vi "RecVOR _Ori.vi"() -> ()   [LabVIEW 2013]
uses:
  <vilib>/userdefined/High Color/IMAQdx.ctl
  <vilib>/vision/Avi1.llb/AviRefnum.ctl
  <vilib>/vision/driver/IMAQdx.llb/IMAQdx Attribute Visibility.ctl
  <vilib>/Instr/_visa.llb/VISA Configure Serial Port (Instr).vi
  <vilib>/DAQmx/read.llb/DAQmx Read (Digital Bool 1Line 1Point).vi
  <vilib>/DAQmx/read.llb/DAQmx Read (Counter U32 1Chan 1Samp).vi
  <vilib>/Utility/file.llb/Write To Spreadsheet File (DBL).vi
  <vilib>/vision/driver/NI_Vision_Acquisition_Software.lvlib
  <resource>/objmgr/imaqdx.rc
  <vilib>/vision/NI_Vision_Development_Module.lvlib
panel:
  in  "Image Flip":u32(ring)=3 items=["Horizontal Flip", "Vertical Flip", "Central Flip", "No Flip"]
  in  "Attribute Name":u32(ring) items=["CameraAttributes::Brightness::Mode", "CameraAttributes::Brightness::Value", "CameraAttributes::Exposure::Mode", "CameraAttributes::Exposure::Value", "CameraAttributes::Gain::Mode", "CameraAttributes::Gain::Value", "CameraAttributes::Gamma::Mode", "CameraAttributes::Gamma::Value", "CameraAttributes::Hue::Mode", "CameraAttributes::Hue::Value", "CameraAttributes::Pan::Mode", "CameraAttributes::Pan::Value", "CameraAttributes::Saturation::Mode", "CameraAttributes::Saturation::Value", "CameraAttributes::Sharpness::Mode", "CameraAttributes::Sharpness::Value", "CameraAttributes::Tilt::Mode", "CameraAttributes::Tilt::Value"]
  in  "Set":bool
  in  "Attribute Value":string
  in  "VISA resource name":refnum<visa-resource-name>="COM3"
  out "Waveform Chart 2":cluster{dbl, dbl}(graph)
  out "Start RecTime":timestamp
  out "Avi Refnum":T1
  out "Elapsed Time":dbl
  out "Frame Num":dbl
  in  "Codec:":string(combo)="Microsoft Video 1"
  out "Rec File Path:":path
  in  "Recording":bool
  in  "Camera Name:":T2="cam0"
  in  "stop":bool
  in  "OpenCam":bool
  out "Frame Rate":dbl(knob) scale=0.0..120.0
  in  "Tab Control":enum32{"Alignment", "Rotator"}(tab)
  out "Alignment":bool
  in  "BCGT":T3={"Brightness"=171.0, "Contrast"=89.0, "Gamma"=2.0, "Threshold_Low"=0.0, "Threshold_High"=255.0} {"Threshold_High" min=0.0 max=255.0 step=1.0 scale=0.0..255.0; "Threshold_Low" min=0 max=255 step=1 scale=0.0..255.0 scale format="%.2f"; "Gamma" min=0.1 max=10 step=0.01 scale=0.1..10.0 scale format="%.1f"; "Contrast" min=1 max=89 step=0.1 scale=0.0..89.0 scale format="%.2f"; "Brightness" min=0 max=255 step=1 scale=0.0..255.0 scale format="%.2f"}
  out "Number of Particles":i32
  out "Distances":sgl[](array[numeric]) format="%.4f"
  out "Array":cluster{"Numeric":dbl, "Numeric":dbl}[](array[cluster])
  out "Image 2":T4(plugin-control)
  out "Degree/sec":dbl(knob) scale=-105.0..105.0
  out "EMST":bool
  out "SVON":bool=TRUE
  in  "Select Mode":T5(ring)
  out "Received Data":string
  out "Transmit Data":string
  in  "Sent":bool
  in  "task/channels in":refnum<k21>="position"
  in  "task/channels in 2":refnum<k21>="dir"
  in  "task/channels in 3":refnum<k21>="dir_vel"
  out "Angle Position":dbl(knob)
  in  "Listbox":i32(listbox)
  in  "Add":bool
  in  "Time":dbl
  in  "Stop":bool
  out "Image":T4(plugin-control)
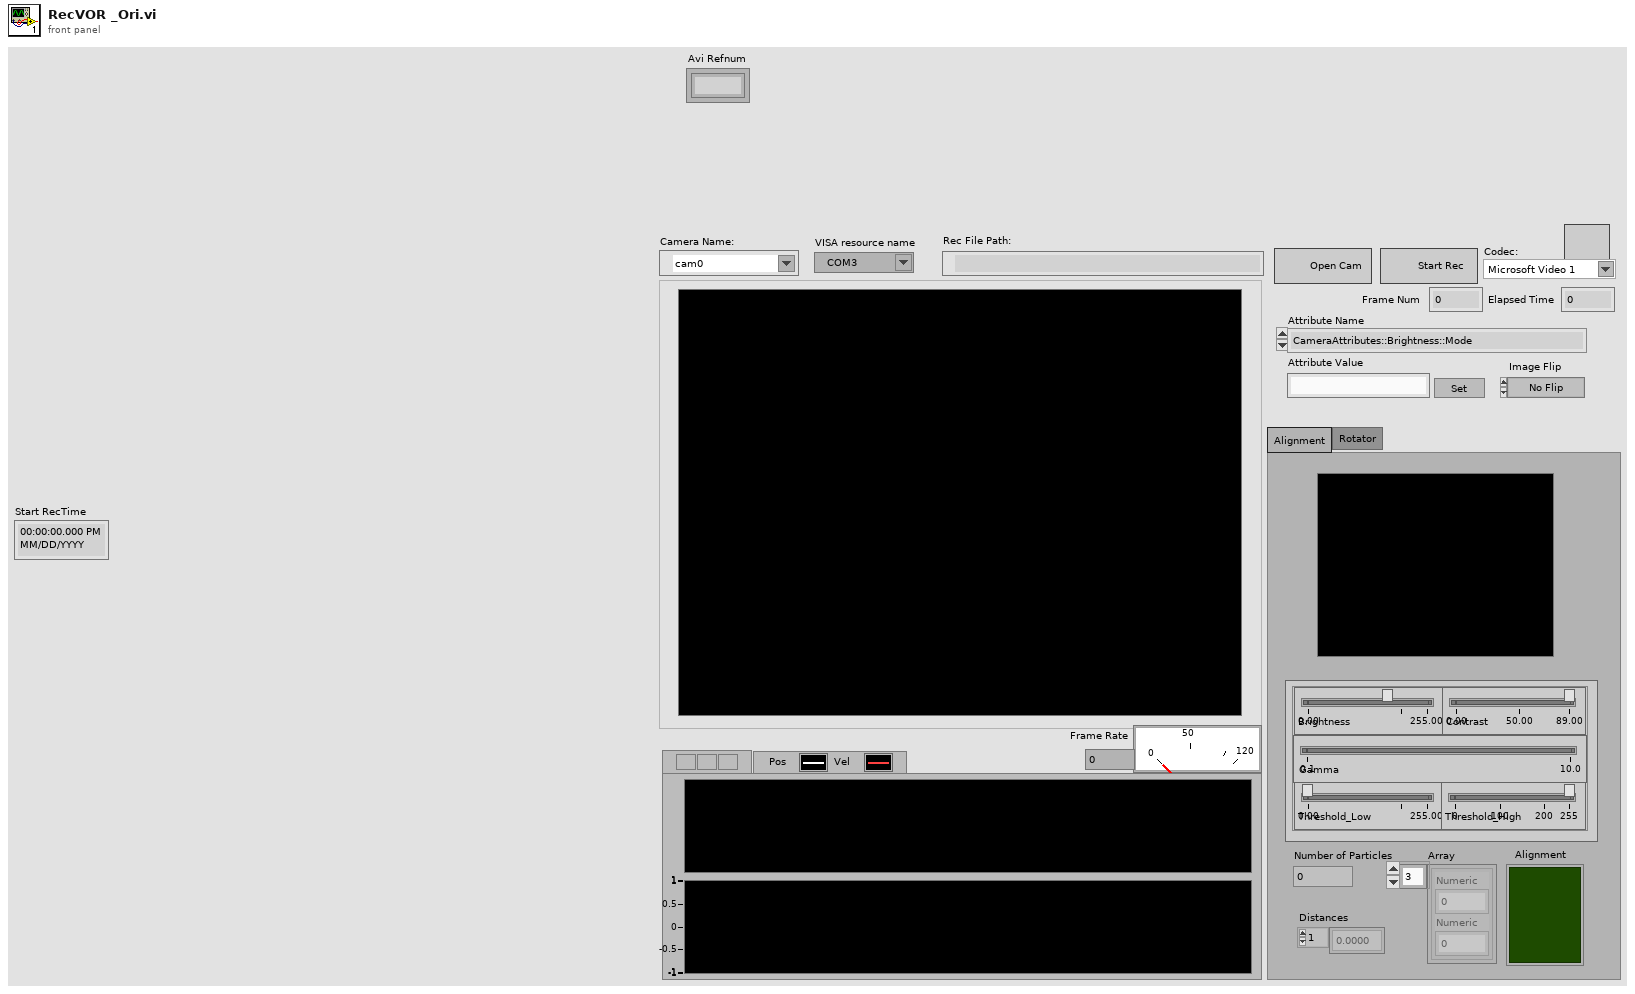
[diagram p1: front panel]
types:
  T1 = typedef "AviRefnum.ctl" = refnum<k1>
  T2 = typedef "IMAQdx.ctl" = refnum<k21>
  T3 = cluster{"Brightness":sgl, "Contrast":sgl, "Gamma":sgl, "Threshold_Low":sgl, "Threshold_High":dbl}
  T4 = typedef "IMAQ Image.ctl" = refnum<image>
  T5 = enum16{"SVON OFF", "SVON ON", "EMST OFF", "EMST ON", "15 degree, 0.1Hz", "15 degree, 0.2Hz", "15 degree, 0.5Hz", "15 degree, 1Hz", "15 degree, 2Hz", "15 degree, 4Hz", "15 degree, 6Hz", "15 degree, 8Hz", "15 degree, 10Hz", "30 degree, 0.1Hz", "30 degree, 0.2Hz", "30 degree, 0.5Hz", "30 degree, 1Hz", "30 degree, 2Hz", "30 degree, 4Hz", "30 degree, 6Hz", "30 degree, 8Hz", "30 degree, 10Hz", "60 degree, 0.1Hz", "60 degree, 0.2Hz", "60 degree, 0.5Hz", "60 degree, 1Hz", "60 degree, 2Hz", "60 degree, 4Hz", "60 degree, 6Hz", "60 degree, 8Hz", "100 degree, 0.1Hz", "100 degree, 0.2Hz", "100 degree, 0.5Hz", "100 degree, 1Hz"}
  T6 = enum8{"Enabled", "Disabled", "Disabled and Grayed Out"}
  T7 = enum16{"Calvar3Open", "CalDataOpen", "CalGrpOpen", "AddAvg", "RmvAvg", "CalCalvar", "AddVar", "SaveVar", "Up", "Dn", "Del"}
  T8 = typedef "NI_Vision_Acquisition_Software.lvlib/IMAQdx Attribute Visibility.ctl" = enum32{"Simple", "Intermediate", "Advanced"}
  T9 = typedef "NI_Vision_Acquisition_Software.lvlib/IMAQdx Attribute Type.ctl" = enum32{"U32", "I64", "DBL", "String", "Enum", "Bool", "Command"}
  T10 = cluster{"Attribute Type":T9, "Readable":bool, "Writable":bool, "Attribute Name":string}[]
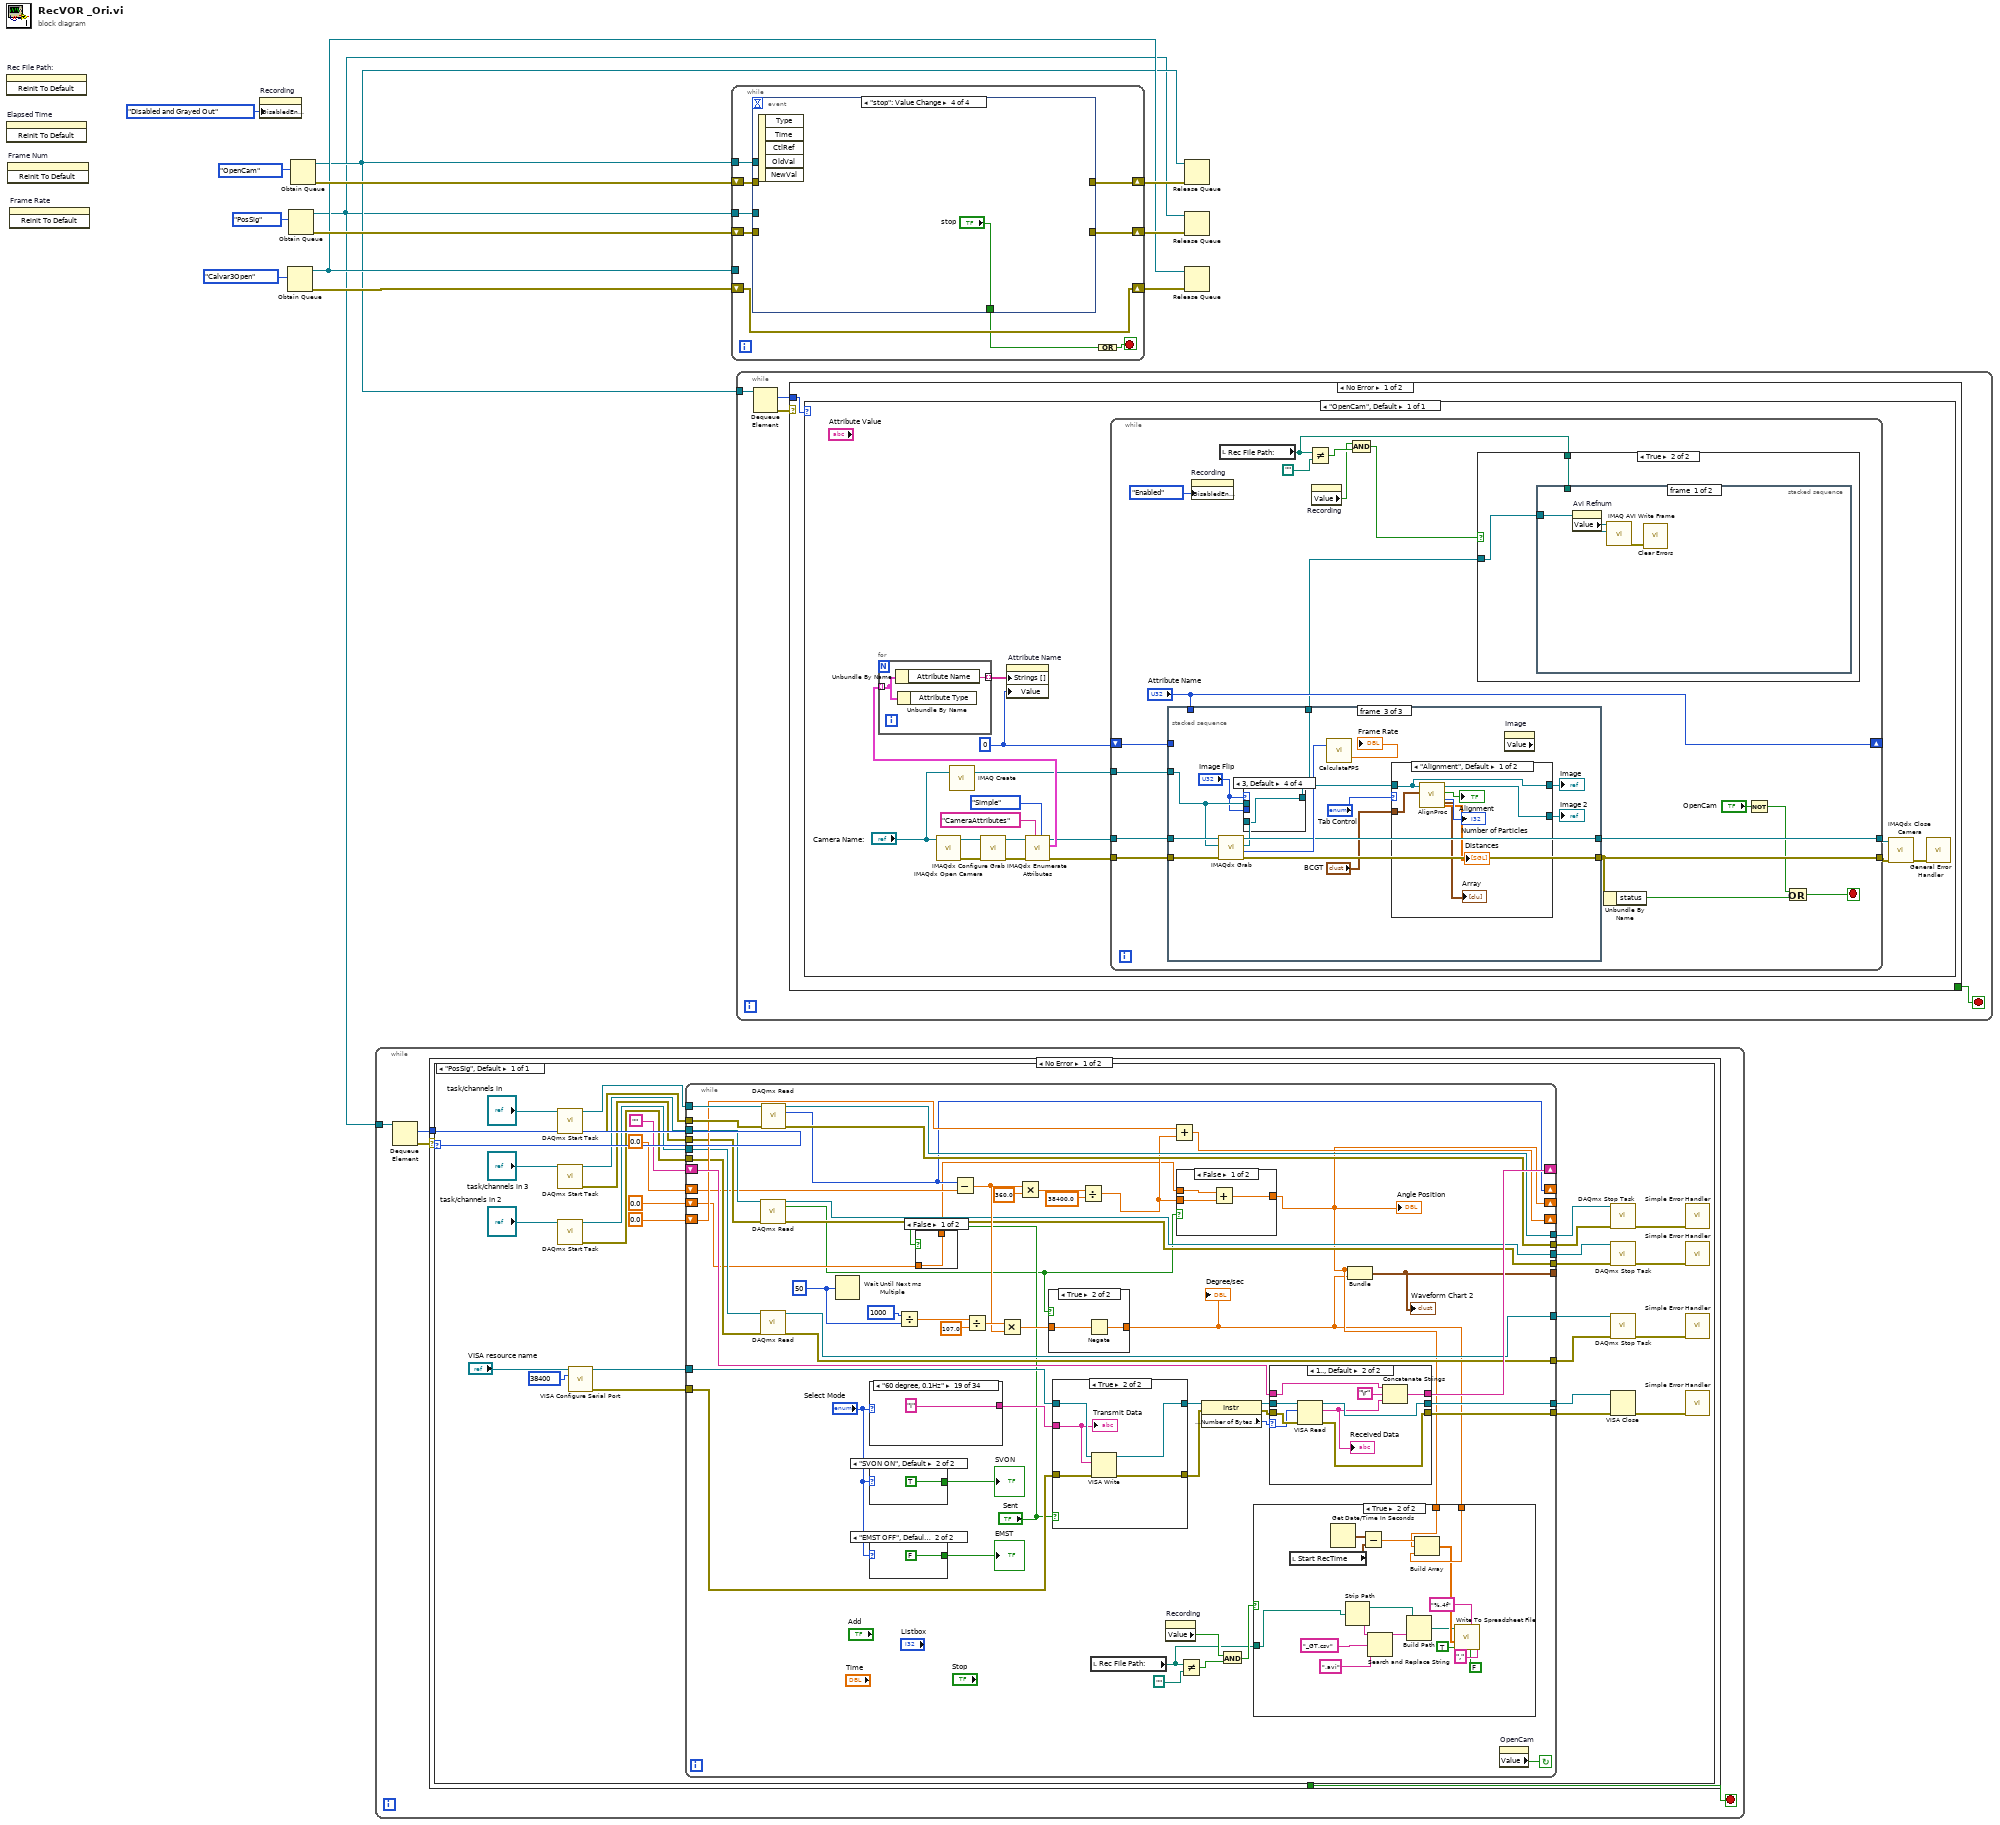
[diagram p0: block diagram]
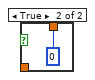
[diagram p3: hidden frame]
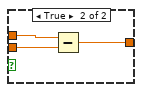
[diagram p5: hidden frame]
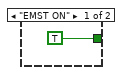
[diagram p6: hidden frame]
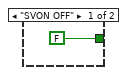
[diagram p7: hidden frame]
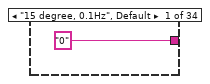
[diagram p8: hidden frame]
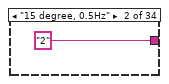
[diagram p9: hidden frame]
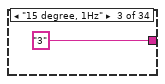
[diagram p10: hidden frame]
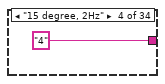
[diagram p11: hidden frame]
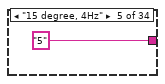
[diagram p12: hidden frame]
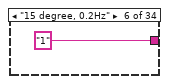
[diagram p13: hidden frame]
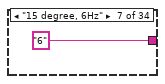
[diagram p14: hidden frame]
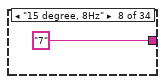
[diagram p15: hidden frame]
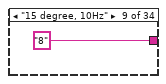
[diagram p16: hidden frame]
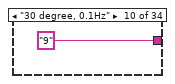
[diagram p17: hidden frame]
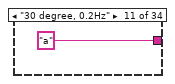
[diagram p18: hidden frame]
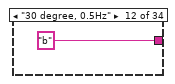
[diagram p19: hidden frame]
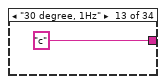
[diagram p20: hidden frame]
diagram:
  n1 = invoke on="Rec File Path:" class="Path" method="Reinit To Default"() -> ()  [unwired: 3 in, 3 out]
  n2 = invoke on="Elapsed Time" class="DigNum (strict)" method="Reinit To Default"() -> ()  [unwired: 3 in, 3 out]
  n3 = invoke on="Frame Num" class="DigNum (strict)" method="Reinit To Default"() -> ()  [unwired: 3 in, 3 out]
  n4 = invoke on="Frame Rate" class="Knob (strict)" method="Reinit To Default"() -> ()  [unwired: 3 in, 3 out]
  n5 = property on="Recording" class="Bool (strict)"("DisabledEnum"=T6."Disabled and Grayed Out" ("Disabled")) -> ()  [unwired: 2 in, 2 out]
  n6 = Obtain Queue(element data type=T7."Calvar3Open" ("Enum")) -> (queue out=w4:refnum<queue>, error out=w9:errorcluster)  [unwired: 4 in, 1 out]
  n7 = Obtain Queue(element data type=enum16{"PosSig"}."PosSig" ("Enum")) -> (queue out=w2:refnum<queue>, error out=w10:errorcluster)  [unwired: 4 in, 1 out]
  n8 = Obtain Queue(element data type=enum16{"OpenCam"}."OpenCam" ("Enum")) -> (queue out=w3:refnum<queue>, error out=w12:errorcluster)  [unwired: 4 in, 1 out]
  n9 = while {
    tunnel: w2 -> [w17]
    stop <- w15 stop-if-true
    n10 = Dequeue Element(queue=w17) -> (element=w14:enum16{"PosSig"}, error out=w16:errorcluster)  [unwired: 2 in, 2 out]
    n11 = case shown="No Error" w16 {
      tunnel: [_ TRUE] -> w15
      tunnel: w14 -> [w18 _]
      frame No Error {
        n12 = case shown="\"PosSig\", Default" w18 {
          frame "PosSig", Default {
            n13 = call <vilib>:"DAQmx Start Task.vi"("task/channels in"="task/channels in") -> ("task out"=w40:refnum<k21>, "error out"=w35:errorcluster)  [unwired: 13 in]
            n14 = call <vilib>:"DAQmx Start Task.vi"("task/channels in"="task/channels in 3") -> ("task out"=w24:refnum<k21>, "error out"=w23:errorcluster)  [unwired: 13 in]
            n15 = call <vilib>:"DAQmx Start Task.vi"("task/channels in"="task/channels in 2") -> ("task out"=w31:refnum<k21>, "error out"=w30:errorcluster)  [unwired: 13 in]
            n16 = call-poly "VISA Configure Serial Port"("VISA resource name"="VISA resource name", "baud rate (9600)"=u32 38400) -> ("VISA resource name out"=w44:refnum<visa-resource-name>, "error out"=w43:errorcluster)  [unwired: 12 in]
            n17 = while {
              tunnel: w43 -> [w101]
              tunnel: w44 -> [w102]
              shift-left: "" -> [w93]
              shift-right: [w92] -> _
              tunnel: [w95] -> w46
              tunnel: [w94] -> w47
              tunnel: [w87] -> w41
              tunnel: w40 -> [w86]
              tunnel: w35 -> [w85]
              tunnel: [w84] -> w39
              shift-right: [w75] -> _
              shift-left: 0.0 ("data") -> [w60]
              shift-right: [w74] -> _
              shift-left: 0.0 -> [w80]
              tunnel: w31 -> [w79]
              tunnel: w30 -> [w78]
              tunnel: [w77] -> w29
              tunnel: [w76] -> w28
              shift-right: [w54] -> _
              shift-left: 0.0 -> [w59]
              tunnel: [w56] -> _
              tunnel: w24 -> [w66]
              tunnel: w23 -> [w65]
              tunnel: [w63] -> w21
              tunnel: [w62] -> w20
              stop <- w57 continue-if-true
              w73 = u32 50 ("millisecond multiple")
              n18 = call-poly <vilib>:"DAQmx Read.vi"("task/channels in"=w66, "error in"=w65) -> ("task out"=w62:refnum<k21>, "data"=w55:bool, "error out"=w63:errorcluster)  [unwired: 11 in]
              n19 = call-poly <vilib>:"DAQmx Read.vi"("task/channels in"=w79, "error in"=w78) -> ("task out"=w76:refnum<k21>, "error out"=w77:errorcluster)  [unwired: 11 in, 1 out]
              n20 = call-poly <vilib>:"DAQmx Read.vi"("task/channels in"=w86, "error in"=w85) -> ("task out"=w84:refnum<k21>, "data"=w75:u32, "error out"=w87:errorcluster)  [unwired: 11 in]
              n21 = Wait Until Next ms Multiple(millisecond multiple=w73) -> ()  [unwired: 1 out]
              n22 = case shown="\"60 degree, 0.1Hz\"" "Select Mode" {
                tunnel: ["0" "2" "3" "4" "5" "1" "6" "7" "8" "9" "a" "b" "c" "d" "e" "f" "g" "h" "i" "j" "k" "l" "m" "n" "o" "p" "r" "t" "u" "v" "q" "z" "s" "w"] -> w91
                frame "15 degree, 0.1Hz", Default {
                }
                frame "15 degree, 0.5Hz" {
                }
                frame "15 degree, 1Hz" {
                }
                frame "15 degree, 2Hz" {
                }
                frame "15 degree, 4Hz" {
                }
                frame "15 degree, 0.2Hz" {
                }
                frame "15 degree, 6Hz" {
                }
                frame "15 degree, 8Hz" {
                }
                frame "15 degree, 10Hz" {
                }
                frame "30 degree, 0.1Hz" {
                }
                frame "30 degree, 0.2Hz" {
                }
                frame "30 degree, 0.5Hz" {
                }
                frame "30 degree, 1Hz" {
                }
                frame "30 degree, 2Hz" {
                }
                frame "30 degree, 4Hz" {
                }
                frame "30 degree, 6Hz" {
                }
                frame "30 degree, 8Hz" {
                }
                frame "30 degree, 10Hz" {
                }
                frame "60 degree, 0.1Hz" {
                }
                frame "60 degree, 0.2Hz" {
                }
                frame "60 degree, 0.5Hz" {
                }
                frame "60 degree, 1Hz" {
                }
                frame "60 degree, 2Hz" {
                }
                frame "60 degree, 4Hz" {
                }
                frame "60 degree, 6Hz" {
                }
                frame "60 degree, 8Hz" {
                }
                frame "100 degree, 0.1Hz" {
                }
                frame "100 degree, 0.2Hz" {
                }
                frame "100 degree, 0.5Hz" {
                }
                frame "100 degree, 1Hz" {
                }
                frame "EMST ON" {
                }
                frame "EMST OFF" {
                }
                frame "SVON ON" {
                }
                frame "SVON OFF" {
                }
              }
              n23 = case shown="\"SVON ON\", Default" "Select Mode" {
                tunnel: [FALSE TRUE] -> w90
                frame "SVON OFF" {
                }
                frame "SVON ON", Default {
                }
              }
              "SVON" <- w90
              n24 = case shown="\"EMST OFF\", Default" "Select Mode" {
                tunnel: [TRUE FALSE] -> w89
                frame "EMST ON" {
                }
                frame "EMST OFF", Default {
                }
              }
              "EMST" <- w89
              n25 = Divide(x=u32 1000, y=w73) -> (x/y=w67:dbl)
              n26 = case shown="False" "Sent" {
                tunnel: w59 -> [w120 _]
                tunnel: [w120 0] -> w58
                frame False {
                }
                frame True {
                }
              }
              n27 = Subtract(x=w75, y=w60) -> (x-y=w69:dbl)
              n28 = Divide(x=w67, y=107.0 ("x")) -> (x/y=w71:dbl)
              n29 = Multiply(x=w71, y=w69) -> (x*y=w64:dbl)
              n30 = Multiply(x=w69, y=360.0) -> (x*y=w82:dbl)
              n31 = case shown="True" w55 {
                tunnel: w64 -> [w122 w124]
                tunnel: [w122 w123] -> w53
                frame False {
                }
                frame True {
                  n32 = Negate(x=w124) -> (-x=w123:dbl)
                }
              }
              "Degree/sec" <- w53
              n33 = case shown="True" "Sent" {
                tunnel: w102 -> [w182 w187]
                tunnel: w101 -> [w181 w185]
                tunnel: [w182 w186] -> w100
                tunnel: [w181 w184] -> w99
                tunnel: w91 -> [_ w183]
                frame False {
                }
                frame True {
                  n34 = VISA Write(VISA resource name=w187, write buffer=w183, error in (no error)=w185) -> (VISA resource name out=w186:refnum<visa-resource-name>, error out=w184:errorcluster)  [unwired: 1 out]
                  "Transmit Data" <- w183
                }
              }
              n35 = Divide(x=w82, y=38400.0) -> (x/y=w70:dbl)
              n36 = local read "Rec File Path:"() -> (w48:path)
              n37 = property on="Recording" class="Bool (strict)"() -> ("Value"=w52:bool)  [unwired: 2 in, 2 out]
              n38 = Add(x=w80, y=w70) -> (x+y=w74:dbl)
              n39 = case shown="False" w55 {
                tunnel: w70 -> [w127 w129]
                tunnel: [w126 w128] -> w54
                tunnel: w58 -> [w125 w130]
                frame False {
                  n40 = Add(x=w125, y=w127) -> (x+y=w126:dbl)
                }
                frame True {
                  n41 = Subtract(x=w130, y=w129) -> (x-y=w128:dbl)
                }
              }
              "Angle Position" <- w54
              n42 = Not Equal?(x=w48, y=path "") -> (x != y?=w50:bool)
              n43 = property class="Instr"(reference=w100, error in=w99) -> (reference out=w96:refnum<visa-resource-name>, error out=w97:errorcluster, "Serial Settings:Number of Bytes at Serial Port"=w98:u32)
              n44 = And(x=w52, y=w50) -> (x .and. y?=w49:bool)
              n45 = case shown="True" w49 {
                tunnel: w54 -> [_ w113]
                tunnel: w53 -> [_ w112]
                tunnel: w48 -> [_ w104]
                frame False {
                }
                frame True {
                  n46 = local read "Start RecTime"() -> (w119:timestamp)
                  n47 = Get Date/Time In Seconds() -> (seconds since 1Jan1904=w118:timestamp)
                  n48 = Strip Path(path=w104) -> (stripped path=w106:path, name=w107:string)
                  n49 = Subtract(x=w118, y=w119) -> (x-y=w114:dbl)
                  n50 = Search and Replace String(input string=w107, search string=".avi", replace string="_GT.csv" ("replace string (\"\")")) -> (result string=w110:string)  [unwired: 5 in, 3 out]
                  n51 = Build Path(base path=w106, name or relative path=w110) -> (appended path=w105:path)
                  n52 = Build Array(w114, w113, w112) -> (w111:dbl[])
                  n53 = call-poly <vilib>:"Write To Spreadsheet File.vi"("delimiter (\\t)"="," ("delimiter (\\t)"), "transpose? (no:F)"=FALSE, "format (%.3f)"="%.4f", "append to file? (new file:F)"=TRUE, "1D data"=w111, "file path (dialog if empty)"=w105) -> ()  [unwired: 2 in, 1 out]
                }
              }
              n54 = case shown="1.., Default" w98 {
                selector: w98 -> [_ w173]
                tunnel: w97 -> [w170 w177]
                tunnel: w96 -> [w171 w175]
                tunnel: [w170 w176] -> w95
                tunnel: [w171 w174] -> w94
                tunnel: w93 -> [w169 w179]
                tunnel: [w169 w178] -> w92
                frame 0 {
                }
                frame 1.., Default {
                  n55 = VISA Read(VISA resource name=w175, byte count=w173, error in (no error)=w177) -> (VISA resource name out=w174:refnum<visa-resource-name>, read buffer=w172:string, error out=w176:errorcluster)  [unwired: 1 out]
                  "Received Data" <- w172
                  n56 = Concatenate Strings(w179, "\r", w172) -> (w178:string)
                }
              }
              n57 = Bundle(w54, w53) -> (w56:cluster{dbl, dbl})  [unwired: 1 in]
              "Waveform Chart 2" <- w56
              n58 = property on="OpenCam" class="Bool (strict)"() -> ("Value"=w57:bool)  [unwired: 2 in, 2 out]
            }
            n59 = call <vilib>:"DAQmx Stop Task.vi"("task/channels in"=w39, "error in"=w41) -> ("error out"=w34:errorcluster)  [unwired: 12 in, 1 out]
            n60 = call <vilib>:"DAQmx Stop Task.vi"("task/channels in"=w20, "error in"=w21) -> ("error out"=w22:errorcluster)  [unwired: 12 in, 1 out]
            n61 = call <vilib>:"DAQmx Stop Task.vi"("task/channels in"=w28, "error in"=w29) -> ("error out"=w27:errorcluster)  [unwired: 12 in, 1 out]
            n62 = VISA Close(VISA resource name=w47, error in (no error)=w46) -> (error out=w38:errorcluster)
            n63 = call <vilib>:"Simple Error Handler.vi"("error in (no error)"=w34) -> ()  [unwired: 4 in, 5 out]
            n64 = call <vilib>:"Simple Error Handler.vi"("error in (no error)"=w22) -> ()  [unwired: 4 in, 5 out]
            n65 = call <vilib>:"Simple Error Handler.vi"("error in (no error)"=w27) -> ()  [unwired: 4 in, 5 out]
            n66 = call <vilib>:"Simple Error Handler.vi"("error in (no error)"=w38) -> ()  [unwired: 4 in, 5 out]
          }
        }
      }
      frame Error {
      }
    }
  }
  n67 = while {
    shift-right: [w195] -> w13
    shift-left: w12 -> [w196]
    tunnel: w3 -> [w197]
    shift-right: [w192] -> w8
    shift-left: w10 -> [w193]
    tunnel: w2 -> [w194]
    tunnel: w4 -> [_]
    shift-right: [w190] -> w7
    shift-left: w9 -> [w190]
    stop <- w191 stop-if-true
    n68 = event shown="[3] \"stop\": Value Change" {
      selector: _ -> [_ _ _ _]
      dyn-events: _ -> [_ _ _ _]
      timeout: _ -> [_ _ _ _]
      tunnel: w197 -> [_ w205 _ _]
      tunnel: w196 -> [_ w204 _ _]
      tunnel: [_ w202 _ _] -> w195
      tunnel: w194 -> [_ w201 _ _]
      tunnel: w193 -> [_ w200 _ _]
      tunnel: [_ w198 _ _] -> w192
      tunnel: [_ _ _ "stop"] -> w189
      event Timeout {
        n69 = event-data() -> ()  [unwired: 1 in, 2 out]
      }
      event "OpenCam": Value Change {
        n70 = event-data() -> ()  [unwired: 1 in, 1 out]
        n71 = Enqueue Element(queue=w205, element=enum16{"OpenCam"}."OpenCam" ("Enum"), error in (no error)=w204) -> (error out=w202:errorcluster)  [unwired: 1 in, 2 out]
        n72 = Enqueue Element(queue=w201, element=enum16{"PosSig"}."PosSig" ("Enum"), error in (no error)=w200) -> (error out=w198:errorcluster)  [unwired: 1 in, 2 out]
      }
      event "Recording": Value Change {
        n73 = event-data() -> ()  [unwired: 1 in, 5 out]
        n74 = case shown="True" "Recording" {
          frame False {
            n75 = property on="Avi Refnum" class="TypRef (strict)"() -> ("Value"=w208:T1)  [unwired: 2 in, 2 out]
            n76 = call "IMAQ AVI Close"("Avi Refnum"=w208) -> ("error out"=w207:errorcluster)  [unwired: 10 in]
            n77 = call <vilib>:"General Error Handler.vi"("error in (no error)"=w207) -> ()  [unwired: 2 in, 13 out]
          }
          frame True {
            n78 = stacked-sequence {
              frame #0 {
                n79 = local read "Frame Rate"() -> (w214:dbl)
                n80 = call "File Dialog"("pattern (all files)"="*.avi") -> ("selected path"=w212:path)  [unwired: 11 in, 3 out]
                "Rec File Path:" <- w212
                n81 = call "IMAQ AVI Create"("Compression Filter"="Codec:", "Frames Per Second"=w214, "AVI Path"=w212) -> ("Avi Refnum"=→"Avi Refnum":T1)  [unwired: 7 in, 1 out]
                n82 = property on="OpenCam" class="Bool (strict)"("DisabledEnum"=T6."Disabled and Grayed Out" ("Disabled")) -> ()  [unwired: 2 in, 2 out]
              }
              frame #1 {
                n83 = local read "Rec File Path:"() -> (w217:path)
                n84 = Strip Path(path=w217) -> (stripped path=w225:path, name=w226:string)
                n85 = Strip Path(path=w217) -> (stripped path=w222:path, name=w221:string)
                n86 = Search and Replace String(input string=w226, search string=".avi", replace string="_VT.csv" ("replace string (\"\")")) -> (result string=w229:string)  [unwired: 5 in, 3 out]
                n87 = Search and Replace String(input string=w221, search string=".avi", replace string="_GT.csv" ("replace string (\"\")")) -> (result string=w218:string)  [unwired: 5 in, 3 out]
                n88 = Build Path(base path=w225, name or relative path=w229) -> (appended path=w224:path)
                n89 = Build Path(base path=w222, name or relative path=w218) -> (appended path=w215:path)
                n90 = call-poly <vilib>:"Write To Spreadsheet File.vi"("delimiter (\\t)"="," ("delimiter (\\t)"), "file path (dialog if empty)"=w224) -> ()  [unwired: 6 in, 1 out]
                n91 = call-poly <vilib>:"Write To Spreadsheet File.vi"("delimiter (\\t)"="," ("delimiter (\\t)"), "file path (dialog if empty)"=w215) -> ()  [unwired: 6 in, 1 out]
              }
              frame #2 {
                n92 = Get Date/Time In Seconds() -> (seconds since 1Jan1904=→"Start RecTime":timestamp)
                "Frame Num" <- 0.0 ("Frame Num")
                "Elapsed Time" <- 0.0 ("Elapsed Time")
              }
            }
          }
        }
      }
      event "stop": Value Change {
        n93 = event-data() -> ()  [unwired: 1 in, 5 out]
      }
    }
    n94 = Compound Arithmetic op=OR(w189) -> (w191:bool)
  }
  n95 = while {
    tunnel: w3 -> [w237]
    stop <- w235 stop-if-true
    n96 = Dequeue Element(queue=w237) -> (element=w234:enum16{"OpenCam"}, error out=w236:errorcluster)  [unwired: 2 in, 2 out]
    n97 = case shown="No Error" w236 {
      tunnel: [_ TRUE] -> w235
      tunnel: w234 -> [w238 _]
      frame No Error {
        n98 = case shown="\"OpenCam\", Default" w238 {
          frame "OpenCam", Default {
            w246 = u32 0 ("BufferInterval")
            n99 = call <vilib>:"IMAQdx Open Camera.vi"("Session In"="Camera Name:") -> ("error out"=w254:errorcluster, "Session Out"=w253:T2)  [unwired: 2 in, 7 out]
            n100 = call "IMAQ Create"("Image Name"="Camera Name:") -> ("New Image"=w243:T4)  [unwired: 3 in, 2 out]
            n101 = call <vilib>:"IMAQdx Configure Grab.vi"("error in"=w254, "Session In"=w253) -> ("error out"=w251:errorcluster, "Session Out"=w252:T2)  [unwired: 8 out]
            n102 = call <vilib>:"IMAQdx Enumerate Attributes.vi"("Visibility"=IMAQdx_Attribute_Visibility."Simple", "Root"="CameraAttributes", "error in"=w251, "Session In"=w252) -> ("error out"=w244:errorcluster, "Attribute Information Array"=w248:T10, "Session Out"=w245:T2)  [unwired: 5 out]
            n103 = for {
              tunnel: w248 -> [w255] mode=indexing
              tunnel: [w256] -> w247 mode=indexing
              n104 = Unbundle By Name(w255) -> ("Attribute Name"=w256:string)
              n105 = Unbundle By Name(w255) -> ()  [unwired: 1 out]
            }
            n106 = property on="Attribute Name" class="Ring (strict)"("Strings []"=w247, "Value"=w246) -> ()  [unwired: 2 in, 2 out]
            n107 = while {
              shift-right: ["Attribute Name"] -> _
              shift-left: w246 -> [w267]
              tunnel: [w265] -> w240
              tunnel: [w264] -> w241
              tunnel: w245 -> [w263]
              tunnel: w244 -> [w262]
              tunnel: w243 -> [w261]
              stop <- w257 stop-if-true
              n108 = stacked-sequence {
                tunnel: w262 -> [w277 w299 w319]
                tunnel: w263 -> [w278 w298 w318]
                tunnel: w267 -> [w281 _ _]
                tunnel: "Attribute Name" -> [w280 _ _]
                tunnel: [_ _ w317] -> w265
                tunnel: [_ _ w316] -> w264
                tunnel: w261 -> [_ _ w313]
                tunnel: [_ _ w310] -> w260
                frame #0 {
                  n109 = Not Equal?(x=w280, y=w281) -> (x != y?=w279:bool)
                  n110 = First Call?() -> (First Call?: T/F=w275:bool)
                  n111 = Or(x=w279, y=w275) -> (x .or. y?=w276:bool)
                  n112 = case shown="True" w276 {
                    tunnel: w278 -> [_ w284]
                    tunnel: w277 -> [_ w283]
                    frame False {
                    }
                    frame True {
                      n113 = property on="Attribute Name" class="Ring (strict)"() -> ("Ring Text.Text"=w289:string)  [unwired: 2 in, 2 out]
                      n114 = property class="IMAQdx"(reference=w284, error in=w283, "Camera Attributes:Active Attribute"=w289) -> (error out=w282:errorcluster, "Camera Attributes:Is Readable"=w288:bool, "Camera Attributes:Is Writable"=w297:bool, "Camera Attributes:Value:String"=w287:string)  [unwired: 1 out]
                      n115 = And(x=w288, y=w297) -> (x .and. y?=w293:bool)
                      n116 = call <vilib>:"Clear Errors.vi"("error in (no error)"=w282) -> ()  [unwired: 6 in, 1 out]
                      n117 = Select(t=0, s=w293, f=2) -> (s? t:f=w292:i32)
                      n118 = Select(t=0, s=w297, f=2) -> (s? t:f=w296:i32)
                      n119 = Select(t=w287, s=w288, f="") -> (s? t:f=w286:string)
                      n120 = property on="Attribute Value" class="Str"("Disabled"=w292) -> ()  [unwired: 2 in, 2 out]
                      n121 = property on="Set" class="Bool"("Disabled"=w296) -> ()  [unwired: 2 in, 2 out]
                      n122 = property on="Attribute Value" class="Str"("Value"=w286) -> ()  [unwired: 2 in, 2 out]
                    }
                  }
                }
                frame #1 {
                  n123 = case shown="True" "Set" {
                    tunnel: w299 -> [_ w302]
                    tunnel: w298 -> [_ w301]
                    frame False {
                    }
                    frame True {
                      n124 = property on="Attribute Name" class="Ring (strict)"() -> ("Ring Text.Text"=w303:string)  [unwired: 2 in, 2 out]
                      n125 = property on="Attribute Value" class="Str"() -> ("Value"=w304:string)  [unwired: 2 in, 2 out]
                      n126 = property class="IMAQdx"(reference=w301, error in=w302, "Camera Attributes:Active Attribute"=w303, "Camera Attributes:Value:String"=w304) -> (error out=w306:errorcluster, "Camera Attributes:Value:String"=w305:string)  [unwired: 1 out]
                      n127 = property on="Attribute Value" class="Str"("Value"=w305) -> ()  [unwired: 2 in, 2 out]
                      n128 = call <vilib>:"Simple Error Handler.vi"("error in (no error)"=w306) -> ()  [unwired: 1 in, 8 out]
                    }
                  }
                }
                frame #2 {
                  n129 = call <vilib>:"IMAQdx Grab.vi"("error in"=w319, "Image In"=w313, "Session In"=w318) -> ("error out"=w316:errorcluster, "Buffer Number Out"=w320:u32, "Image Out"=w314:T4, "Session Out"=w317:T2)  [unwired: 1 in, 4 out]
                  n130 = case shown="3, Default" "Image Flip" {
                    tunnel: w314 -> [w330 w336 w339 w341]
                    tunnel: [w329 w335 w337 w341] -> w310
                    tunnel: "Image Flip" -> [w332 w334 w338 _]
                    tunnel: w313 -> [w331 w333 w340 _]
                    frame 0 {
                      n131 = call "IMAQ Symmetry"("Type of Symmetry"=w332, "Image Dst"=w331, "Image Src"=w330) -> ("Image Dst Out"=w329:T4)  [unwired: 2 in, 1 out]
                    }
                    frame 1 {
                      n132 = call "IMAQ Symmetry"("Type of Symmetry"=w334, "Image Dst"=w333, "Image Src"=w336) -> ("Image Dst Out"=w335:T4)  [unwired: 2 in, 1 out]
                    }
                    frame 2 {
                      n133 = call "IMAQ Symmetry"("Type of Symmetry"=w338, "Image Dst"=w340, "Image Src"=w339) -> ("Image Dst Out"=w337:T4)  [unwired: 2 in, 1 out]
                    }
                    frame 3, Default {
                    }
                  }
                  n134 = call "CalculateFPS.vi"("buffer number"=w320) -> ("processed FPS"=→"Frame Rate":dbl)  [unwired: 2 out]
                  n135 = case shown="\"Alignment\", Default" "Tab Control" {
                    tunnel: w310 -> [w322 w328]
                    tunnel: "BCGT" -> [w327 _]
                    tunnel: [w322 w328] -> w308
                    tunnel: [w321 _] -> w307
                    frame "Alignment", Default {
                      n136 = call "AlignProc.vi"("BCGT"=w327, "Img_In"=w322) -> ("Distances"=→"Distances":sgl[], "Number of Particles"=→"Number of Particles":i32, "Boolean"=→"Alignment":bool, "Image Out"=w321:T4, "Array"=→"Array":cluster{"Numeric":dbl, "Numeric":dbl}[])  [unwired: 5 in]
                    }
                    frame "Rotator" {
                    }
                  }
                  "Image 2" <- w307
                  "Image" <- w308
                  n137 = property on="Image" class="ImageControl" props=["Value"]() -> ()  [unwired: 2 in, 3 out]
                }
              }
              n138 = property on="Recording" class="Bool (strict)"("DisabledEnum"=T6."Enabled" ("Disabled")) -> ()  [unwired: 2 in, 2 out]
              n139 = local read "Rec File Path:"() -> (w268:path)
              n140 = Not Equal?(x=w268, y=path "") -> (x != y?=w271:bool)
              n141 = property on="Recording" class="Bool (strict)"() -> ("Value"=w270:bool)  [unwired: 2 in, 2 out]
              n142 = And(x=w270, y=w271) -> (x .and. y?=w269:bool)
              n143 = case shown="True" w269 {
                tunnel: w260 -> [_ w345]
                tunnel: w268 -> [_ w344]
                frame False {
                  w343 = 0.0 ("Frame Num")
                  n144 = property on="OpenCam" class="Bool (strict)"("DisabledEnum"=T6."Enabled" ("Disabled")) -> ()  [unwired: 2 in, 2 out]
                  n145 = local write "Frame Num"(w343) -> ()
                  n146 = local write "Elapsed Time"(w343) -> ()
                }
                frame True {
                  n147 = stacked-sequence {
                    tunnel: w345 -> [w348 _]
                    tunnel: w344 -> [_ w352]
                    frame #0 {
                      n148 = property on="Avi Refnum" class="TypRef (strict)"() -> ("Value"=w347:T1)  [unwired: 2 in, 2 out]
                      n149 = call "IMAQ AVI Write Frame"("Image"=w348, "Avi Refnum"=w347) -> ("error out"=w346:errorcluster)  [unwired: 8 in, 1 out]
                      n150 = call <vilib>:"Clear Errors.vi"("error in (no error)"=w346) -> ()  [unwired: 6 in, 1 out]
                    }
                    frame #1 {
                      n151 = local read "Start RecTime"() -> (w363:timestamp)
                      n152 = local read "Frame Num"() -> (w349:dbl)
                      n153 = Get Date/Time In Seconds() -> (seconds since 1Jan1904=w362:timestamp)
                      n154 = Subtract(x=w362, y=w363) -> (x-y=w351:dbl)
                      n155 = Strip Path(path=w352) -> (stripped path=w354:path, name=w355:string)
                      n156 = Increment(x=w349) -> (x+1=w364:dbl)
                      n157 = Build Array(w351, w349) -> (w350:dbl[])
                      n158 = local write "Elapsed Time"(w351) -> ()
                      n159 = Search and Replace String(input string=w355, search string=".avi", replace string="_VT.csv" ("replace string (\"\")")) -> (result string=w358:string)  [unwired: 5 in, 3 out]
                      n160 = local write "Frame Num"(w364) -> ()
                      n161 = Build Path(base path=w354, name or relative path=w358) -> (appended path=w353:path)
                      n162 = call-poly <vilib>:"Write To Spreadsheet File.vi"("delimiter (\\t)"="," ("delimiter (\\t)"), "transpose? (no:F)"=FALSE, "append to file? (new file:F)"=TRUE, "1D data"=w350, "file path (dialog if empty)"=w353) -> ()  [unwired: 3 in, 1 out]
                    }
                  }
                }
              }
              n163 = Unbundle By Name(w264) -> ("status"=w259:bool)
              n164 = Not(x="OpenCam") -> (.not. x?=w258:bool)
              n165 = Or(x=w258, y=w259) -> (x .or. y?=w257:bool)
            }
            n166 = call <vilib>:"IMAQdx Close Camera.vi"("error in"=w241, "Session In"=w240) -> ("error out"=w239:errorcluster)  [unwired: 9 out]
            n167 = call <vilib>:"General Error Handler.vi"("error in (no error)"=w239) -> ()  [unwired: 2 in, 13 out]
          }
        }
      }
      frame Error {
      }
    }
  }
  n168 = Release Queue(queue=w3, error in (no error)=w13) -> ()  [unwired: 1 in, 3 out]
  n169 = Release Queue(queue=w2, error in (no error)=w8) -> ()  [unwired: 1 in, 3 out]
  n170 = Release Queue(queue=w4, error in (no error)=w7) -> ()  [unwired: 1 in, 3 out]
